vi "GenerateUntriggeredStimulus.vi"(8 "error in (no error)":errorcluster, 11 "FullWormGWN in":refnum<class "FullWormGWN.lvclass">) -> (0 "error out":errorcluster, 2 "UntriggeredStimulusOut":sgl[][](array[numeric]), 3 "FullWormGWN out":refnum<class "FullWormGWN.lvclass">)   [LabVIEW 2019, in "FullWormGWN.lvclass"]
uses:
  FullWormGWN.lvclass
  C:/Users/mochil/Dropbox/LeiferShaevitz/Github/ProjectAPI/LabviewVIs/StimulusObject.lvclass
  StimulusObject.lvclass/StimulusObject.ctl
  FullWormGWN.lvclass/FullWormGWN.ctl
  ParametersGlobal.vi
  <vilib>/ptbypt/Signal Generation.llb/Gaussian White Noise PtByPt.vi
  StimulusObject.lvclass
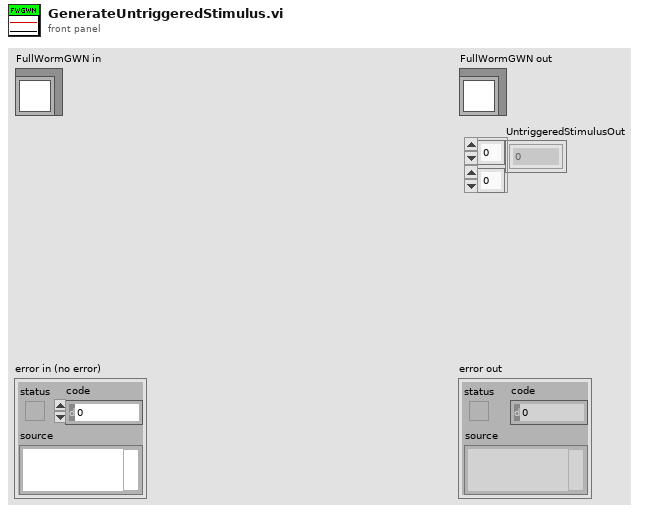
[diagram p1: front panel]
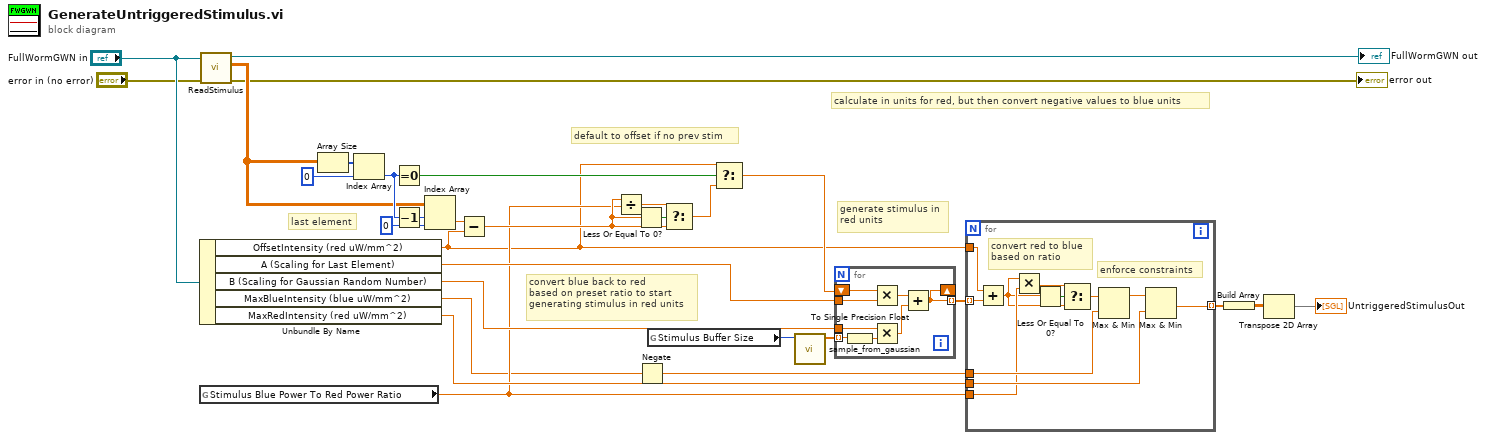
[diagram p0: block diagram]
diagram:
  # "generate stimulus in\nred units"
  # "convert blue back to red\nbased on preset ratio to start\ngenerating stimulus in red units"
  # "calculate in units for red, but then convert negative values to blue units"
  # "default to offset if no prev stim"
  # "last element"
  n1 = Unbundle By Name("FullWormGWN in") -> ("OffsetIntensity (red uW/mm^2)"=w6:sgl, "A (Scaling for Last Element)"=w23:sgl, "B (Scaling for Gaussian Random Number)"=w22:sgl, "MaxBlueIntensity (blue uW/mm^2)"=w15:sgl, "MaxRedIntensity (red uW/mm^2)"=w21:sgl)
  n2 = global read "ParametersGlobal.vi" "Stimulus Blue Power To Red Power Ratio"() -> (w16:sgl)
  n3 = call "ReadStimulus.vi"("error in (no error)"="error in (no error)", "StimulusObject in"="FullWormGWN in") -> ("error out"=→"error out":errorcluster, "StimulusOut"=w17:sgl[][], "StimulusObject out"=→"FullWormGWN out":refnum<class "FullWormGWN.lvclass">)  [unwired: 7 in]
  n4 = Array Size(array=w17) -> (size(s)=w30:i32[])
  n5 = Index Array(array=w30, index=0) -> (element=w25:i32)
  n6 = Equal To 0?(x=w25) -> (x = 0?=w28:bool)
  n7 = Decrement(x=w25) -> (x-1=w24:i32)
  n8 = Index Array(array=w17, index (row)=w24, index (col)=0 ("disabled index (col)")) -> (element=w26:sgl)
  n9 = Subtract(x=w26, y=w6) -> (x-y=w19:sgl)
  n10 = Divide(x=w19, y=w16) -> (x/y=w3:sgl)
  n11 = Less Or Equal To 0?(x=w19) -> (x <= 0?=w4:bool)
  n12 = Negate(x=w15) -> (-x=w14:sgl)
  n13 = global read "ParametersGlobal.vi" "Stimulus Buffer Size"() -> (w20:i32)
  n14 = Select(t=w3, s=w4, f=w19) -> (s? t:f=w18:sgl)
  n15 = Select(t=w6, s=w28, f=w18) -> (s? t:f=w27:sgl)
  n16 = call "sample_from_gaussian.vi"("Samples"=w20) -> ("Output"=w11:dbl[])  [unwired: 10 in]
  n17 = for {
    shift-right: [w31] -> _
    shift-left: w27 -> [w37]
    tunnel: w23 -> [w38]
    tunnel: w22 -> [w34]
    tunnel: w11 -> [w36] mode=indexing
    tunnel: [w31] -> w10 mode=indexing
    n18 = To Single Precision Float(number=w36) -> (single precision float=w35:sgl)
    n19 = Multiply(x=w37, y=w38) -> (x*y=w32:sgl)
    n20 = Multiply(x=w34, y=w35) -> (x*y=w33:sgl)
    n21 = Add(x=w32, y=w33) -> (x+y=w31:sgl)
  }
  n22 = for {
    tunnel: w10 -> [w47] mode=indexing
    tunnel: [w48] -> w2 mode=indexing
    tunnel: w6 -> [w46]
    tunnel: w14 -> [w45]
    tunnel: w21 -> [w44]
    tunnel: w16 -> [w40]
    # "convert red to blue\nbased on ratio"
    # "enforce constraints"
    n23 = Add(x=w46, y=w47) -> (x+y=w39:sgl)
    n24 = Multiply(x=w39, y=w40) -> (x*y=w42:sgl)
    n25 = Less Or Equal To 0?(x=w39) -> (x <= 0?=w43:bool)
    n26 = Select(t=w42, s=w43, f=w39) -> (s? t:f=w41:sgl)
    n27 = Max & Min(x=w41, y=w45) -> (max(x,y)=w49:sgl)  [unwired: 1 out]
    n28 = Max & Min(x=w49, y=w44) -> (min(x,y)=w48:sgl)  [unwired: 1 out]
  }
  n29 = Build Array(w2) -> (w1:sgl[][])
  n30 = Transpose 2D Array(2D array=w1) -> (transposed array=→"UntriggeredStimulusOut":sgl[][])
